vi "destroyPubDataEvents.vi"(8 "error in (no error)":errorcluster, 11 "DataListenerThisComponent in":refnum<class "DataListenerThisComponent.lvclass">) -> (0 "error out":errorcluster, 3 "DataListenerThisComponent out":refnum<class "DataListenerThisComponent.lvclass">)   [LabVIEW 2015]
uses:
  DataListenerThisComponent.lvclass
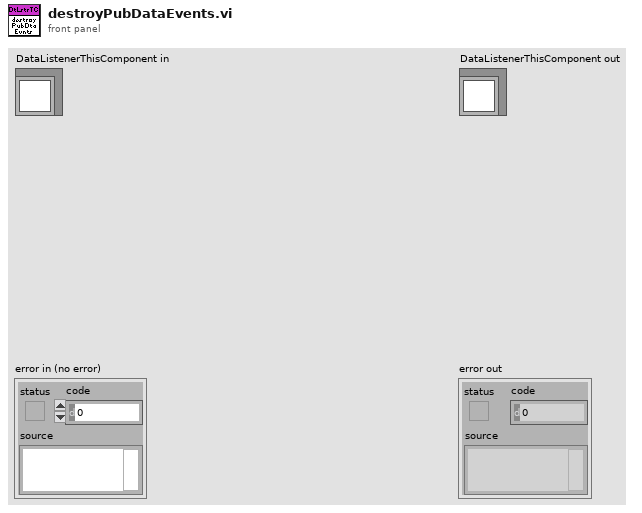
[diagram p1: front panel]
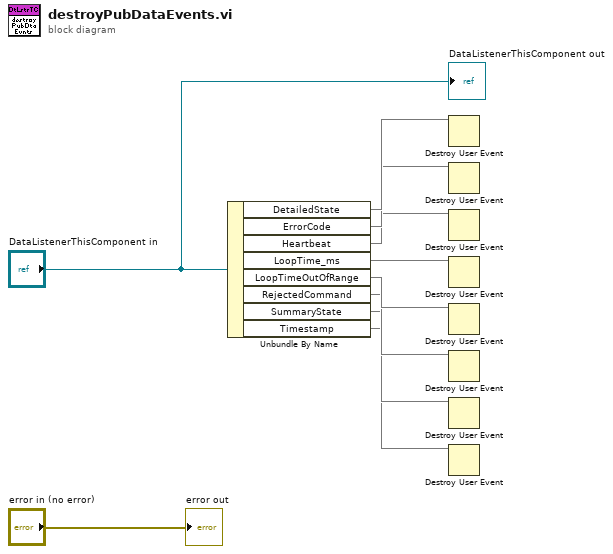
[diagram p0: block diagram]
diagram:
  n1 = Unbundle By Name("DataListenerThisComponent in") -> ("DetailedState"=w9, "ErrorCode"=w8, "Heartbeat"=w7, "LoopTime_ms"=w6, "LoopTimeOutOfRange"=w5, "RejectedCommand"=w4, "SummaryState"=w3, "Timestamp"=w2)
  n2 = Destroy User Event(user event=w9) -> ()  [unwired: 1 in, 1 out]
  n3 = Destroy User Event(user event=w8) -> ()  [unwired: 1 in, 1 out]
  n4 = Destroy User Event(user event=w7) -> ()  [unwired: 1 in, 1 out]
  n5 = Destroy User Event(user event=w6) -> ()  [unwired: 1 in, 1 out]
  n6 = Destroy User Event(user event=w5) -> ()  [unwired: 1 in, 1 out]
  n7 = Destroy User Event(user event=w4) -> ()  [unwired: 1 in, 1 out]
  n8 = Destroy User Event(user event=w3) -> ()  [unwired: 1 in, 1 out]
  n9 = Destroy User Event(user event=w2) -> ()  [unwired: 1 in, 1 out]
  "error out" <- "error in (no error)"
  "DataListenerThisComponent out" <- "DataListenerThisComponent in"
